vi "Init Series Graph.vi"(0 "TG Series Graph in":refnum<class "TG Series Graph.lvclass">, 1 "Z-Chart Ref":refnum<vi>, 2 "Shots":u32, 3 "Z Scale.Marker Values[]":cluster{"Numeric":dbl, "Numeric":u32}[](array[cluster]), 5 "IntGraph Ref":refnum<vi>, 7 "Image Size":cluster{"Height":u32, "Width":u32}, 9 "Y-Graph Ref":refnum<vi>, 11 "error in (no error)":errorcluster, 12 "X-Graph Ref":refnum<vi>) -> (4 "TG Series Graph out":refnum<class "TG Series Graph.lvclass">, 15 "error out":errorcluster)   [LabVIEW 2023, in "TG Series Graph.lvclass"]
uses:
  TG Series Graph.lvclass
  TG Series Graph.lvclass/TG Series Graph.ctl
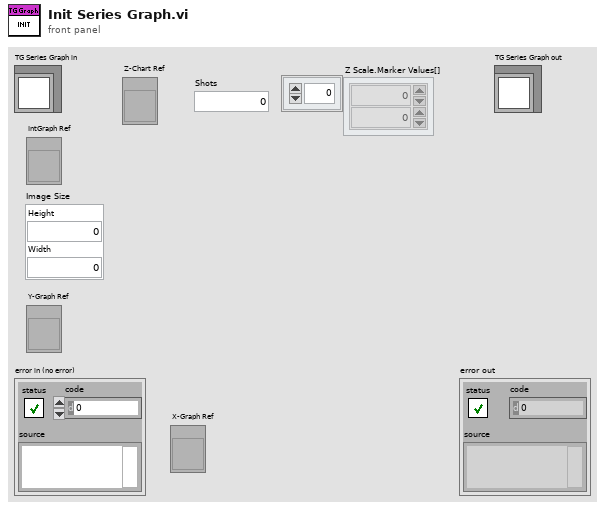
[diagram p1: front panel]
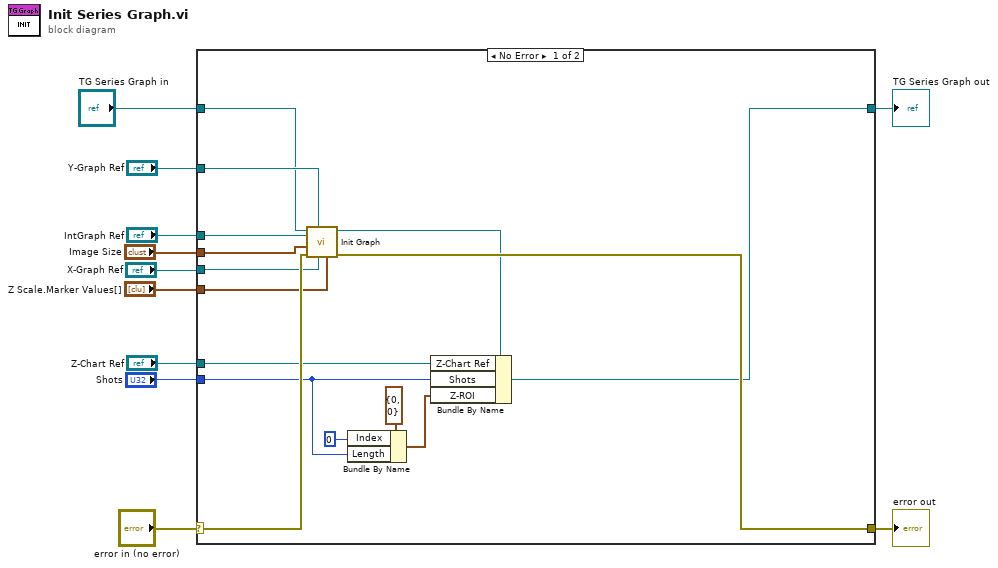
[diagram p0: block diagram]
diagram:
  n1 = case shown="No Error" "error in (no error)" {
    selector: "error in (no error)" -> [w23 w28]
    tunnel: [w22 w28] -> w10
    tunnel: [w12 w27] -> w8
    tunnel: "TG Series Graph in" -> [w21 w27]
    tunnel: "Y-Graph Ref" -> [w25 _]
    tunnel: "IntGraph Ref" -> [w26 _]
    tunnel: "Image Size" -> [w24 _]
    tunnel: "Z-Chart Ref" -> [w20 _]
    tunnel: "X-Graph Ref" -> [w19 _]
    tunnel: "Shots" -> [w15 _]
    tunnel: "Z Scale.Marker Values[]" -> [w18 _]
    frame No Error {
      n2 = call-dynamic "Init Graph.vi"("Z Scale.Marker Values[]"=w18, "X-Graph Ref"=w19, "Y-Graph Ref"=w25, "error in (no error)"=w23, "Images Size"=w24, "IntGraph Ref"=w26, "Intensity Graph in"=w21) -> ("error out"=w22:errorcluster, "Intensity Graph out"=w13:refnum<class "TG Series Graph.lvclass">)  [unwired: 3 in]
      n3 = Bundle By Name(cluster=cluster{"Index":u32, "Length":u32} {"Index"=0, "Length"=0} ("Z-ROI"), "Index"=u32 0, "Length"=w15) -> (w14:cluster{"Index":u32, "Length":u32})
      n4 = Bundle By Name(cluster=w13, "Z-Chart Ref"=w20, "Shots"=w15, "Z-ROI"=w14) -> (w12:refnum<class "TG Series Graph.lvclass">)
    }
    frame Error {
    }
  }
  "error out" <- w10
  "TG Series Graph out" <- w8
